vi "PmuErrorHdr.vi"(8 "error in (no error)":errorcluster, 11 "OutputToFile":refnum<class "OutputToFileBasePlugin.lvclass">) -> (0 "error out":errorcluster, 2 "ErrorHdr":string[](array[string]), 3 "OutputToFile":refnum<class "OutputToFileBasePlugin.lvclass">)   [LabVIEW 2017, in "OutputToFilePlugins.lvlib" / "OutputToFileBasePlugin.lvclass"]
uses:
  OutputToFileBasePlugin.lvclass
  OutputToFileBasePlugin.lvclass/OutputToFileBasePlugin.ctl
  Accessors/Read clConfigOptions.vi
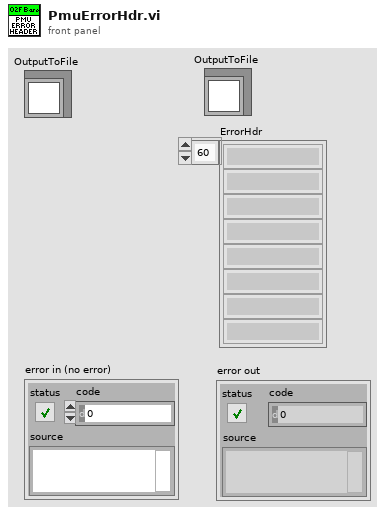
[diagram p1: front panel]
types:
  T1 = typedef "OutputToFilePlugins.lvlib/OutputToFileBasePlugin.lvclass/PmuCfgOpt.ctl" = cluster{"TIME_BASE":u64, "STN":string, "IDCODE":u16, "rdoPolRect":enum32{"Rectangular", "Polar"}, "rdoFloatInt":enum32{"Float", "Integer"}, "PHUNIT":u64, "rdoFreqDfreq":enum32{"Float", "Integer"}, "CHNAM":string[], "chkCfg2Prefix":bool}
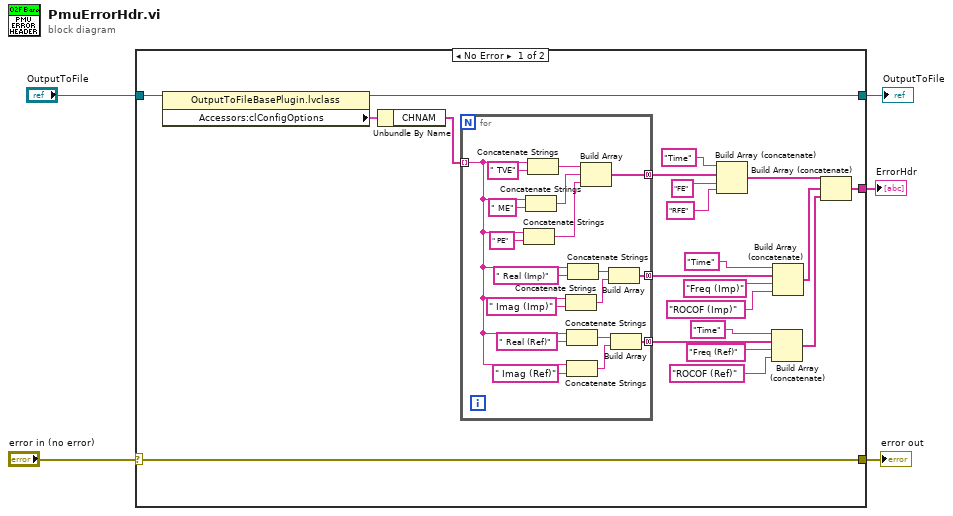
[diagram p0: block diagram]
diagram:
  n1 = case shown="No Error" "error in (no error)" {
    selector: "error in (no error)" -> [w19 w46]
    tunnel: [w19 w46] -> w4
    tunnel: "OutputToFile" -> [w26 w45]
    tunnel: [w24 w45] -> w2
    tunnel: [w12 _] -> w1
    frame No Error {
      n2 = property class="OutputToFileBasePlugin.lvclass"(reference=w26) -> (reference out=w24:refnum<class "OutputToFileBasePlugin.lvclass">, "Accessors:clConfigOptions"=w25:T1)  [unwired: 1 in, 1 out]
      n3 = Unbundle By Name(w25) -> ("CHNAM"=w23:string[])
      n4 = for {
        tunnel: w23 -> [w32] mode=indexing
        tunnel: [w38] -> w22 mode=concatenating
        tunnel: [w33] -> w18 mode=concatenating
        tunnel: [w27] -> w15 mode=concatenating
        n5 = Concatenate Strings(w32, " PE" ("string")) -> (w39:string)
        n6 = Concatenate Strings(w32, " ME" ("string")) -> (w40:string)
        n7 = Concatenate Strings(w32, " TVE" ("string")) -> (w41:string)
        n8 = Concatenate Strings(w32, " Imag (Imp)" ("string")) -> (w34:string)
        n9 = Concatenate Strings(w32, " Real (Ref)" ("string")) -> (w29:string)
        n10 = Concatenate Strings(w32, " Imag (Ref)" ("string")) -> (w28:string)
        n11 = Concatenate Strings(w32, " Real (Imp)" ("string")) -> (w35:string)
        n12 = Build Array(w41, w40, w39) -> (w38:string[])
        n13 = Build Array(w35, w34) -> (w33:string[])
        n14 = Build Array(w29, w28) -> (w27:string[])
      }
      n15 = Build Array (concatenate)("Time" ("string"), w22, "FE" ("string"), "RFE" ("string")) -> (w11:string[])
      n16 = Build Array (concatenate)("Time" ("string"), w15, "Freq (Ref)" ("string"), "ROCOF (Ref)" ("string")) -> (w9:string[])
      n17 = Build Array (concatenate)("Time" ("string"), w18, "Freq (Imp)" ("string"), "ROCOF (Imp)" ("string")) -> (w10:string[])
      n18 = Build Array (concatenate)(w11, w10, w9) -> (w12:string[])
    }
    frame Error {
    }
  }
  "error out" <- w4
  "OutputToFile" <- w2
  "ErrorHdr" <- w1
